vi "Pcre2SubstringFromSubjectByOffsets (ba).vi"(9 "OffsetPastMatch":i32, 10 "MatchOffset":i32, 11 "Subject":string) -> (1 "AfterSubstring":string, 3 "BeforeSubstring":string)   [LabVIEW 2021, in "libpcre2-8.lvlib"]
uses:
  libpcre2-8.lvlib
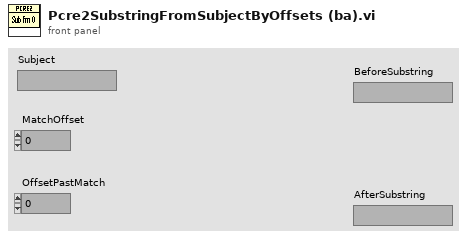
[diagram p1: front panel]
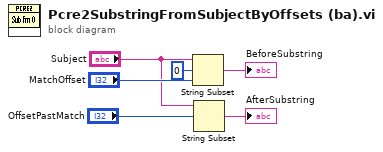
[diagram p0: block diagram]
diagram:
  n1 = String Subset(string="Subject", offset (0)=0, length (rest)="MatchOffset") -> (substring=→"BeforeSubstring":string)
  n2 = String Subset(string="Subject", offset (0)="OffsetPastMatch") -> (substring=→"AfterSubstring":string)  [unwired: 1 in]
